vi "6240AData_terrminate.vi"(8 "error in (no error)":errorcluster, 11 "6240AData in":refnum<class "6240AData.lvclass">) -> (0 "error out":errorcluster, 3 "6240AData out":refnum<class "6240AData.lvclass">)   [LabVIEW 2017, in "6240AData.lvclass"]
uses:
  6240AData.lvclass
  6240AData.lvclass/6240AData.ctl
  istr.lib/ADCMT 6240/ADCMT 6240.lvlib
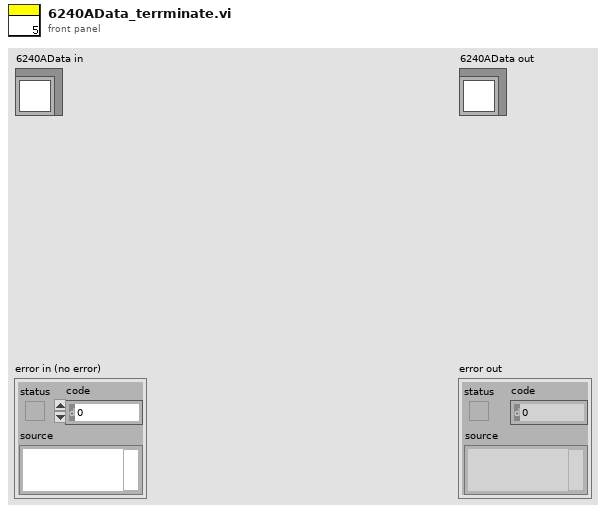
[diagram p1: front panel]
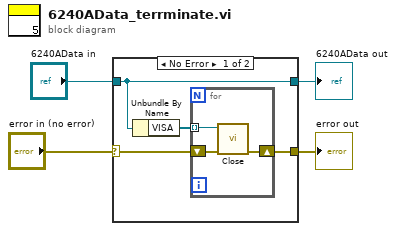
[diagram p0: block diagram]
diagram:
  n1 = case shown="No Error" "error in (no error)" {
    selector: "error in (no error)" -> [w6 w13]
    tunnel: [w5 w13] -> w3
    tunnel: [w8 w12] -> w1
    tunnel: "6240AData in" -> [w8 w12]
    frame No Error {
      n2 = Unbundle By Name(w8) -> ("VISA"=w7:refnum<visa-resource-name>[])
      n3 = for {
        tunnel: w7 -> [w11] mode=indexing
        shift-right: [w9] -> w5
        shift-left: w6 -> [w10]
        n4 = call "Close.vi"("error in (no error)"=w10, "VISA resource name"=w11) -> ("error out"=w9:errorcluster)  [unwired: 9 in]
      }
    }
    frame Error {
    }
  }
  "error out" <- w3
  "6240AData out" <- w1
